vi "SP Convert Format Item to String.vi"(7 "Format":T1 items=["Log Mag", "Phase", "Expanded Phase", "Delay", "Smith", "Polar", "Lin Mag", "SWR", "Loss", "Real", "Imaginary"]) -> (3 "Format String":string)   [LabVIEW 2011]
uses:
  TypeDefs/SP Display Format.ctl
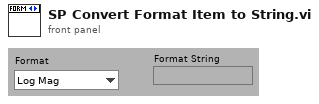
[diagram p1: front panel]
types:
  T1 = typedef "SP Display Format.ctl" = i32
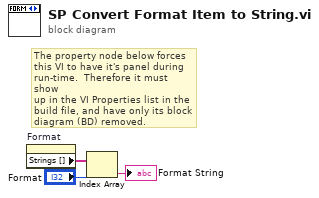
[diagram p0: block diagram]
diagram:
  # "The property node below forces\nthis VI to have it's panel during\nrun-time.  Therefore it must show\nup in the VI Properties list in the\nbuild file, and have only its block\ndiagram (BD) removed."
  n1 = property on="Format" class="Ring (strict)"() -> ("Strings []"=w3:string[])  [unwired: 2 in, 2 out]
  n2 = Index Array(array=w3, index="Format") -> (element=→"Format String":string)
